vi "dialog.vi"(0 "Enable":bool=TRUE, 1 "Strasse":string, 5 "error in (no error)":errorcluster) -> (14 "Breite":u8 caption="String")   [LabVIEW 2019]
doc: "Displays a standard dialog box that prompts users to enter information, such as a user name and password.\n--------------------\n\nThis Express VI is configured as follows:\n\nMessage to Display to the User:Strassenbreite\nThe inputs are: \nNumber: Breite"
panel:
  in  "Breite cm":u8 caption="String"
  out "error out":errorcluster
  in  "Cancel":bool
  in  "OK2":bool
  out "OK":bool
  in  "OK1":bool
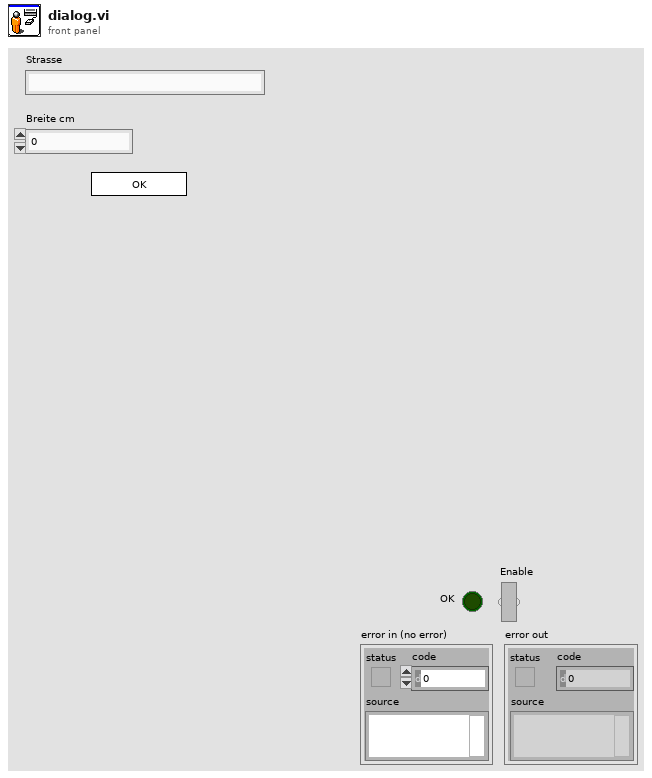
[diagram p1: front panel]
types:
  T1 = cluster{"Input Name":string, "Input Data Type":i32}[]
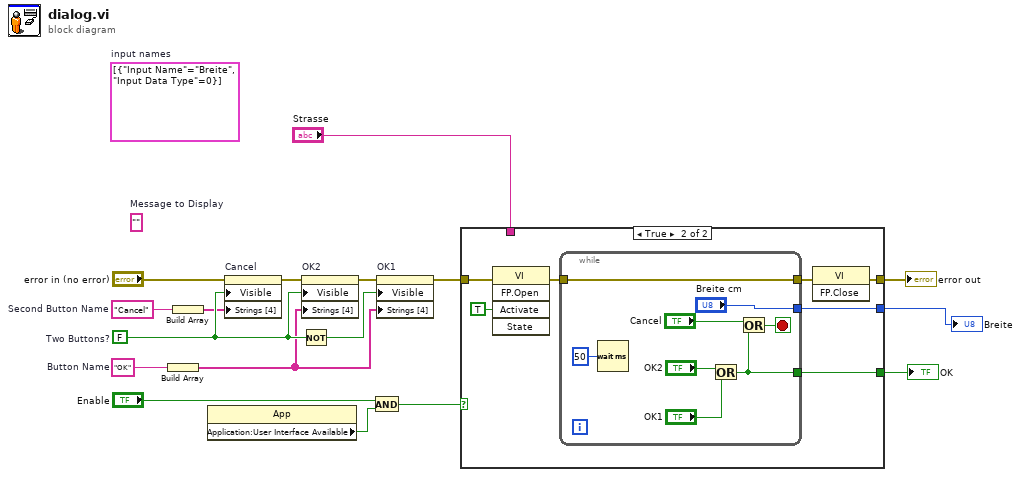
[diagram p0: block diagram]
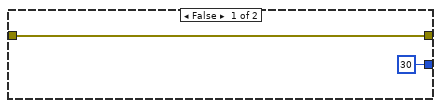
[diagram p2: hidden frame]
diagram:
  (unwired) T1 [{"Input Name"="Breite", "Input Data Type"=0}]  # input names
  w11 = "Cancel"  # Second Button Name
  w9 = "OK"  # Button Name
  (unwired) ""  # Message to Display
  w17 = FALSE  # Two Buttons?
  n1 = Build Array(w9) -> (w10:string[])
  n2 = Build Array(w11) -> (w12:string[])
  n3 = property class="App"() -> ("Application:User Interface Available"=w4:bool)  [unwired: 2 in, 2 out]
  n4 = property on="Cancel" class="Bool"(error in="error in (no error)", "Visible"=w17, "Strings [4]"=w12) -> (error out=w14:errorcluster)  [unwired: 1 in, 1 out]
  n5 = Not(x=w17) -> (.not. x?=w15:bool)
  n6 = property on="OK2" class="Bool"(error in=w14, "Visible"=w17, "Strings [4]"=w10) -> (error out=w13:errorcluster)  [unwired: 1 in, 1 out]
  n7 = And(x="Enable", y=w4) -> (x .and. y?=w3:bool)
  n8 = property on="OK1" class="Bool"(error in=w13, "Visible"=w15, "Strings [4]"=w10) -> (error out=w8:errorcluster)  [unwired: 1 in, 1 out]
  n9 = case shown="True" w3 {
    tunnel: [_ w26] -> w16
    tunnel: w8 -> [w19 w25]
    tunnel: [w19 w24] -> w6
    tunnel: [u8 30 ("Breite 2") w20] -> w2
    tunnel: "Strasse" -> [_ _]
    frame False {
    }
    frame True {
      n10 = invoke class="VI" method="FP.Open"(error in=w25, "Activate"=TRUE ("Activate?")) -> (error out=w22:errorcluster)  [unwired: 3 in, 4 out]
      n11 = while "Main While Loop" {
        tunnel: [w31] -> w26
        tunnel: w22 -> [w28]
        tunnel: [w28] -> w21
        tunnel: ["Breite cm"] -> w20
        stop <- w29 stop-if-true
        n12 = Wait (ms)(milliseconds to wait=u32 50 ("millisecond multiple")) -> ()  [unwired: 1 out]
        n13 = Or(x="OK2", y="OK1") -> (x .or. y?=w31:bool)
        n14 = Or(x="Cancel", y=w31) -> (x .or. y?=w29:bool)
      }
      n15 = invoke class="VI" method="FP.Close"(error in=w21) -> (error out=w24:errorcluster)  [unwired: 2 in, 2 out]
    }
  }
  "OK" <- w16
  "error out" <- w6
  "Breite" <- w2
